vi "WzNetRem_Global.vi"() -> ()   [LabVIEW 2012, in "Wizzler_RemoteTK.lvlib" / "Wizzler_NetworkRemoteToolkit.lvlib"]
uses:
  Wizzler_NetworkRemoteToolkit.lvlib
panel:
  in  "ProcessRAWdata_SRSI":refnum<vi>
  out "Measurement DATA Ref":refnum<vi>
  in  "GetSpectroSettings":refnum<vi>
  in  "SetSpectroSettings":refnum<vi>
  out "Localhost?":bool
  in  "GetEnumDescs":refnum<vi>
  in  "GetStatus":refnum<vi>
  in  "ChangeFeedbackMode":refnum<vi>
  out "ResultReceiver_Daemon":refnum<vi>
  in  "SwitchRunButton":refnum<vi>
  in  "ChangeAlgorithm":refnum<vi>
  in  "LockGUI":refnum<vi>
  in  "GetIDs":refnum<vi>
  in  "Wizzler App Ref":refnum<vi>
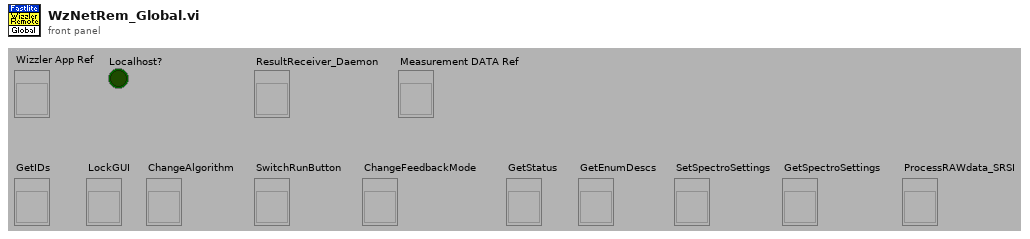
[diagram p1: front panel]
diagram:
